vi "Topcon GPS.vi"   [LabVIEW 2011]
uses:
  _GlobalVariables&Libraries/ATV Program Global Variables.vi
types:
  T1 = cluster{"GPS VISA resource name":refnum<visa-resource-name>, "GPS Error":errorcluster, "Disable GPS VISA":bool, "Latitude":dbl, "Longitude":dbl, "Latitude Uncertainty":dbl, "Longitude Uncertainty":dbl, "GPS Signal":u32}
  T2 = cluster{"End ATV Program":bool, "E-Stop":bool, "Save Logfile":bool, "Logfile Iteration Delay (ms)":u32, "Loop iteration time (ms)":u32, "Logfile Location":path, "Default GPS Navigation Path":path, "Computer":string, "Default GPS Boundary Path":path}
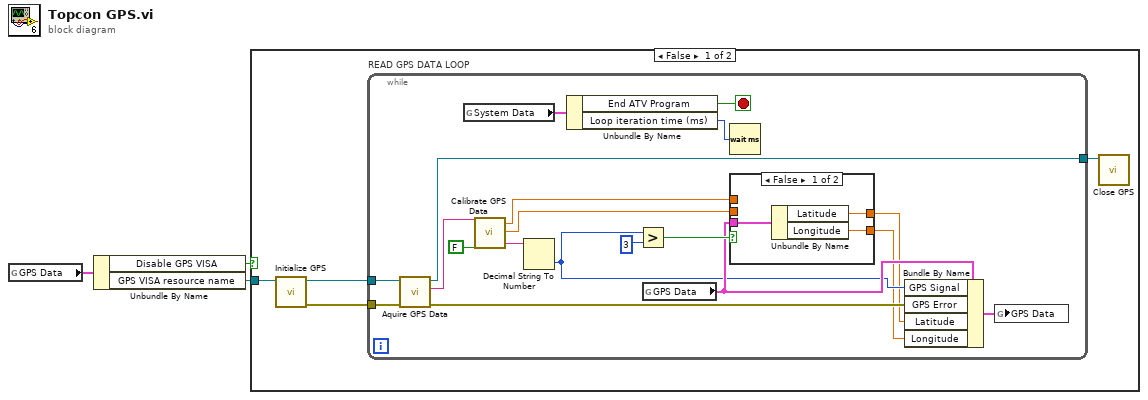
[diagram p0: block diagram]
diagram:
  n1 = global read "ATV Program Global Variables.vi" "GPS Data"() -> (w3:T1)
  n2 = Unbundle By Name(w3) -> ("Disable GPS VISA"=w2:bool, "GPS VISA resource name"=w1:refnum<visa-resource-name>)
  n3 = case shown="False" w2 {
    tunnel: w1 -> [w4 _]
    frame False {
      n4 = call "Initialize GPS.vi"("VISA resource name"=w4) -> ("error out"=w5:errorcluster, "VISA resource name out"=w6:refnum<visa-resource-name>)  [unwired: 9 in]
      n5 = while "READ GPS DATA LOOP" {
        tunnel: [w13] -> w7
        tunnel: w6 -> [w12]
        tunnel: w5 -> [w11]
        stop <- w14 stop-if-true
        n6 = call "Aquire GPS Data.vi"("error in"=w11, "VISA resource name in"=w12) -> ("error out"=w17:errorcluster, "read buffer"=w26:string, "VISA resource name out"=w13:refnum<visa-resource-name>)  [unwired: 7 in]
        n7 = global read "ATV Program Global Variables.vi" "System Data"() -> (w16:T2)
        n8 = call "Calibrate GPS Data.vi"("Read Buffer"=w26, "Calibrate"=FALSE) -> ("Latitude"=w25:dbl, "Longitude"=w24:dbl, "Satellites Tracked"=w23:string)  [unwired: 18 in, 5 out]
        n9 = Decimal String To Number(string=w23) -> (number=w18:i32)  [unwired: 2 in, 1 out]
        n10 = Unbundle By Name(w16) -> ("End ATV Program"=w14:bool, "Loop iteration time (ms)"=w15:u32)
        n11 = Greater?(x=w18, y=3) -> (0:w21:bool)
        n12 = global read "ATV Program Global Variables.vi" "GPS Data"() -> (w19:T1)
        n13 = Wait (ms)(milliseconds to wait=w15) -> ()  [unwired: 1 out]
        n14 = case shown="False" w21 {
          tunnel: w19 -> [w29 _]
          tunnel: w25 -> [_ w31]
          tunnel: w24 -> [_ w30]
          tunnel: [w28 w31] -> w10
          tunnel: [w27 w30] -> w9
          frame False {
            n15 = Unbundle By Name(w29) -> ("Latitude"=w28:dbl, "Longitude"=w27:dbl)
          }
          frame True {
          }
        }
        n16 = Bundle By Name(cluster=w19, "GPS Signal"=w18, "GPS Error"=w17, "Latitude"=w10, "Longitude"=w9) -> (w20:T1)
        n17 = global write "ATV Program Global Variables.vi" "GPS Data"(w20) -> ()
      }
      n18 = call "Close GPS.vi"("VISA resource name"=w7) -> ()  [unwired: 10 in, 1 out]
    }
    frame True {
    }
  }
